vi "Read RT1.vi"(8 "error in (no error)":errorcluster, 11 "Remote Terminal in":refnum<class "Remote Terminal.lvclass">) -> (0 "error out":errorcluster, 2 "RT1":bool, 3 "Remote Terminal out":refnum<class "Remote Terminal.lvclass">)   [LabVIEW 2016, in "BCI-1553 API.lvlib" / "Remote Terminal.lvclass"]
doc: "Return a flag indicating if this current Remote Terminal is setup as the first or second Remote Terminal on the module."
uses:
  Remote Terminal.lvclass
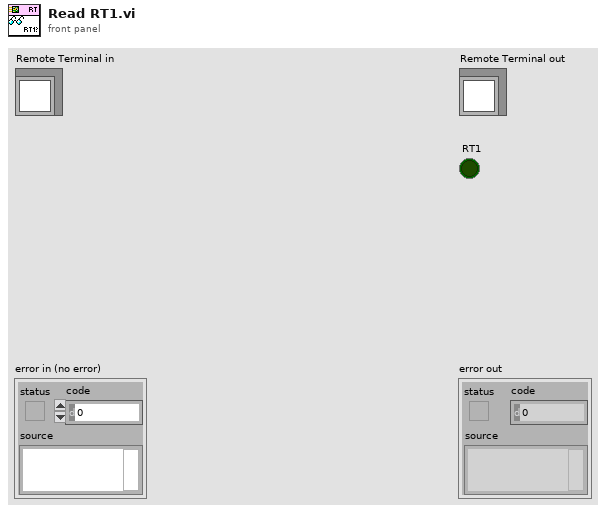
[diagram p1: front panel]
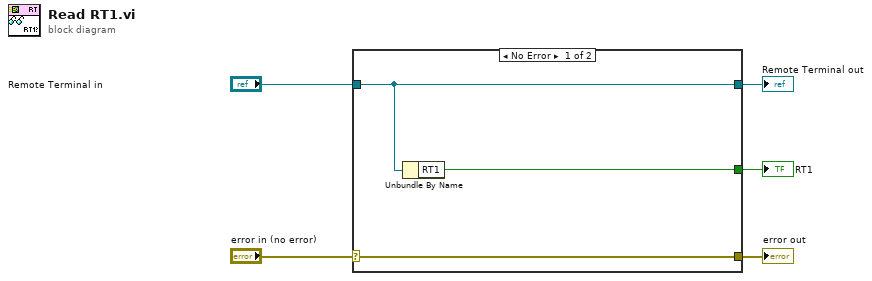
[diagram p0: block diagram]
diagram:
  n1 = case shown="No Error" "error in (no error)" {
    selector: "error in (no error)" -> [w8 w9]
    tunnel: [w8 w9] -> w4
    tunnel: [w7 w10] -> w2
    tunnel: "Remote Terminal in" -> [w7 w10]
    tunnel: [w6 _] -> w1
    frame No Error {
      n2 = Unbundle By Name(w7) -> ("RT1"=w6:bool)
    }
    frame Error {
    }
  }
  "error out" <- w4
  "Remote Terminal out" <- w2
  "RT1" <- w1
